vi "DEV test VIs wrapped.vi"() -> ()   [LabVIEW 2018, in "Image Management.lvlib"]
uses:
  Image Management.lvlib
  receipt parsing/Receipt Parsing.lvlib
  database/Items--cluster.ctl
  database/Database.lvlib
  database/Purchased_Items--cluster.ctl
  database/Visits--cluster.ctl
panel:
  out "TotalPrice":dbl
  out "Unit":string[](array[string])
  out "NumberOfUnits":dbl[](array[numeric])
  out "TaxStatus":string[](array[string])
  out "PrintedNames":string[](array[string])
  out "Prices":string[](array[string])
  out "Items":string[](array[string])
  out "Footer":string[](array[string])
  out "Header":string[](array[string])
  out "Main Body":string[](array[string])
  out "Image 2":T1(plugin-control)
  out "Array":string[](array[string])
  out "Columns (Pixels)":i32
  out "Rows (Pixels)":i32
  out "Image":T1(plugin-control)
  out "Rows Where Whitespace Starts":i32[](array[numeric])
  out "Image Pixels (I16)":i16[][](array[numeric])
  out "Error Out":errorcluster
  in  "Error In":errorcluster
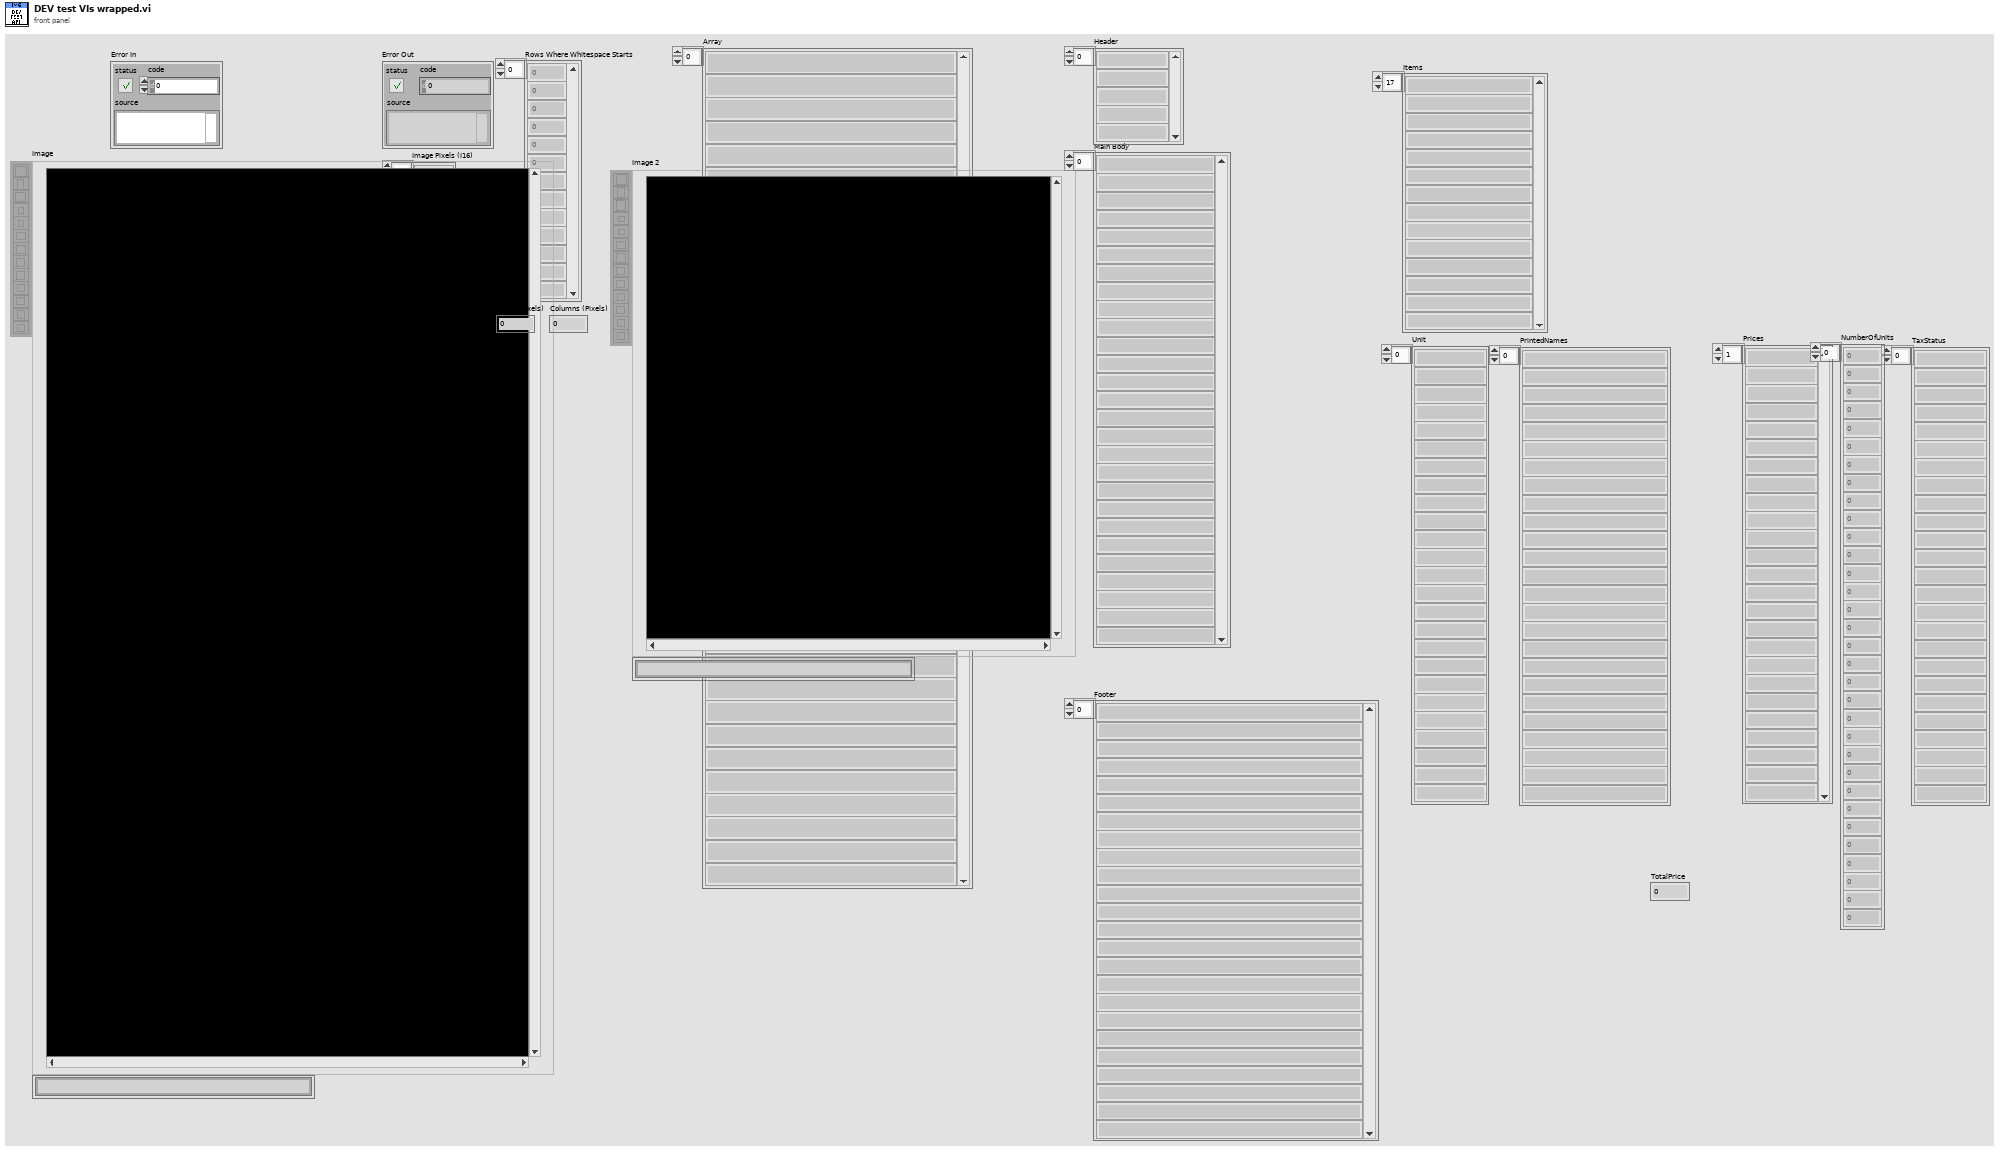
[diagram p1: front panel]
types:
  T1 = typedef "IMAQ Image.ctl" = refnum<image>
  T2 = typedef "Database.lvlib/Visits--cluster.ctl" = cluster{"Timestamp":timestamp, "TotalSpend":dbl, "SpendTaxedA":dbl, "SpendTaxedB":dbl, "Location":string, "NumberOfItems":i32, "NumberOfUniqueItems":i32, "TotalDiscount":dbl, "ReceiptImagePath":string}
  T3 = typedef "Database.lvlib/Purchased_Items--cluster.ctl" = cluster{"ItemName":string, "TotalPriceIncludingDiscount":dbl, "NumberOfUnits":i32, "VisitID":i32, "TotalDiscount":dbl}
  T4 = typedef "Database.lvlib/Items--cluster.ctl" = cluster{"ItemName":string, "PrintedNames":string, "TaxStatus":string, "Unit":string, "IsFood":bool, "IsVeg":bool, "IsFavourite":bool}
  T5 = typedef "ROI Descriptor" = cluster{"Global Rectangle":i32[], "Contours":cluster{"ID":enum32{"External", "Internal"}, "Type":u32, "Coordinates":i32[]}[]}
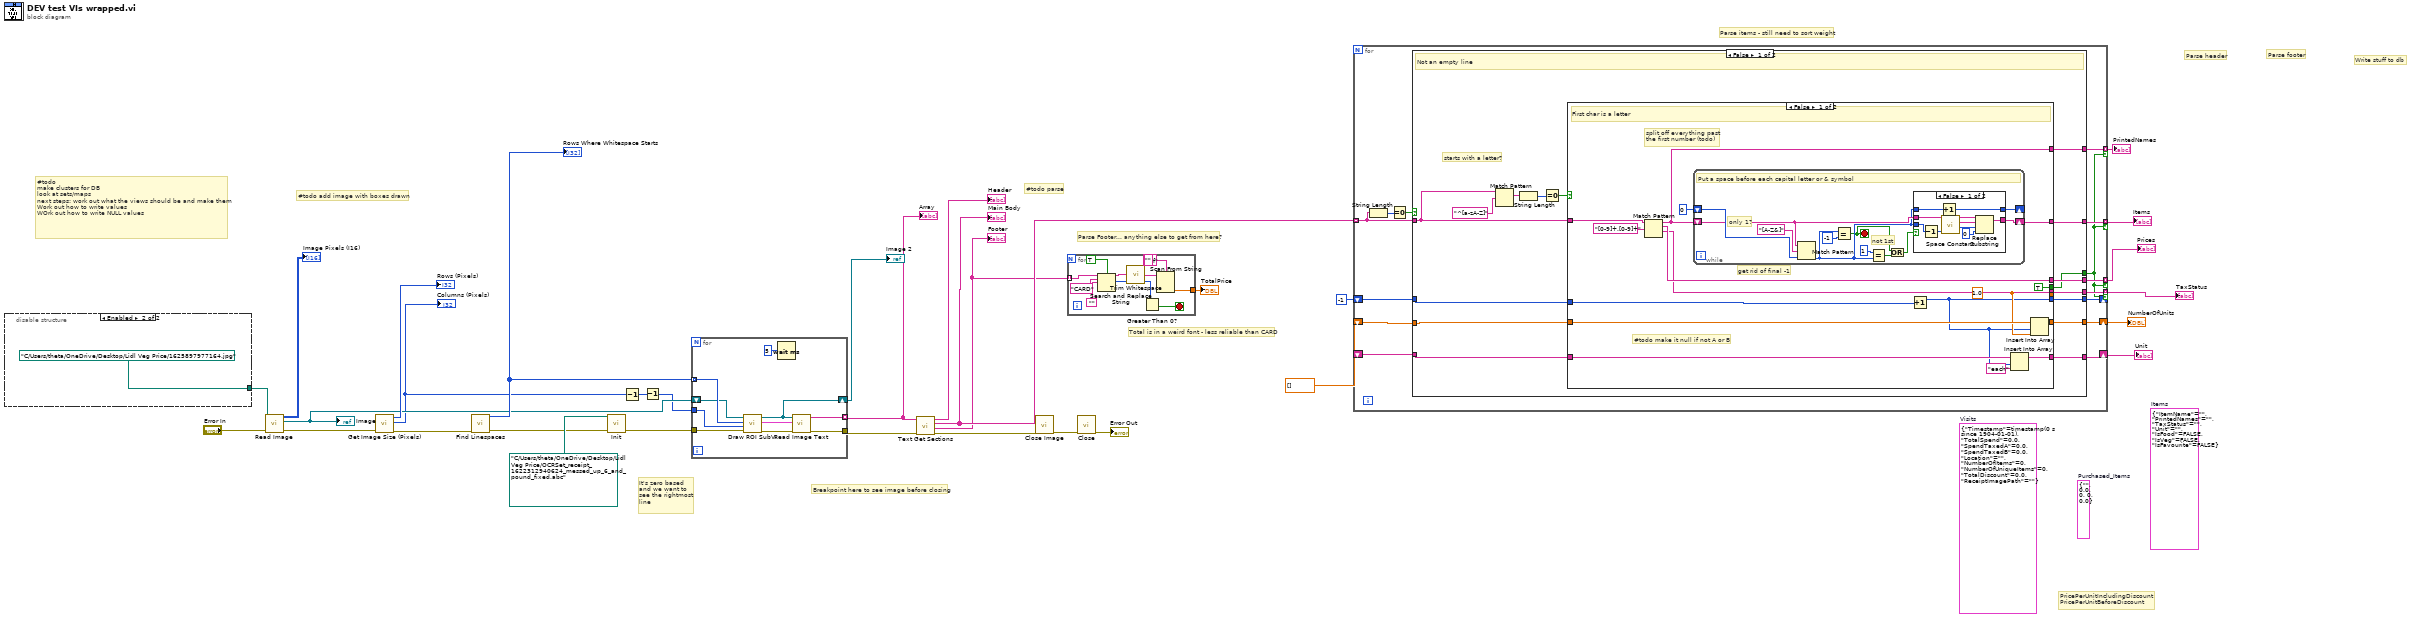
[diagram p0: block diagram]
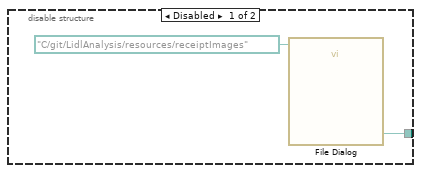
[diagram p2: hidden frame]
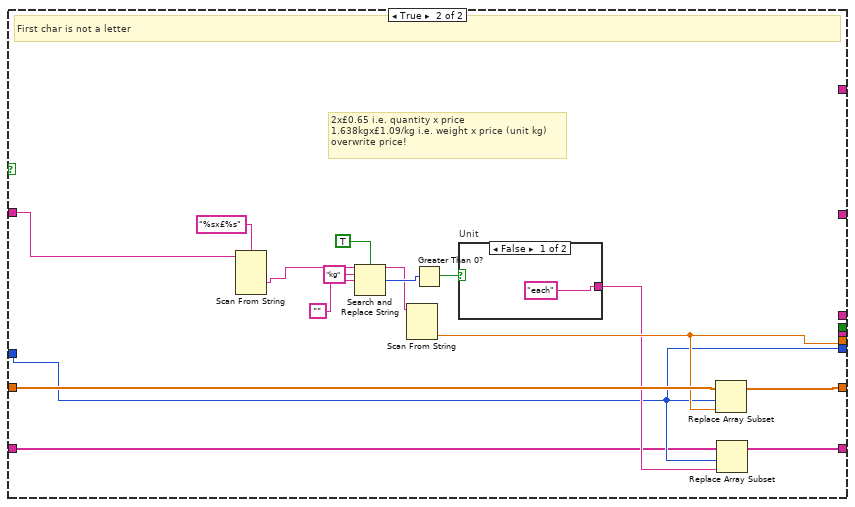
[diagram p4: hidden frame]
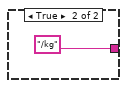
[diagram p5: hidden frame]
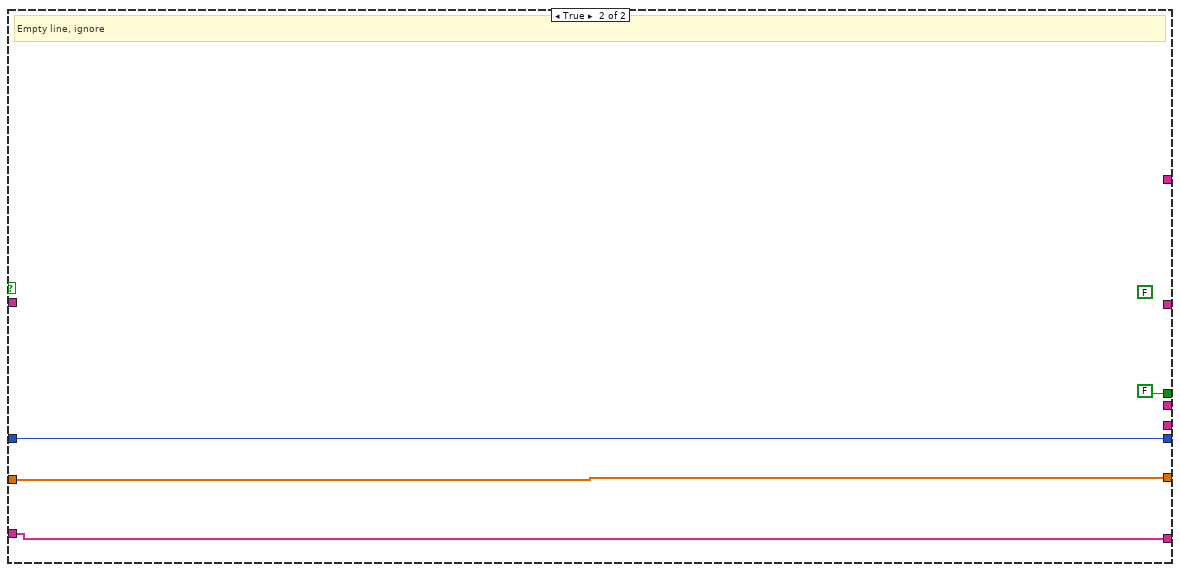
[diagram p6: hidden frame]
diagram:
  (unwired) T2 {"Timestamp"=timestamp(0 s since 1904-01-01), "TotalSpend"=0.0, "SpendTaxedA"=0.0, "SpendTaxedB"=0.0, "Location"="", "NumberOfItems"=0, "NumberOfUniqueItems"=0, "TotalDiscount"=0.0, "ReceiptImagePath"=""}  # Visits
  (unwired) T3 {"ItemName"="", "TotalPriceIncludingDiscount"=0.0, "NumberOfUnits"=0, "VisitID"=0, "TotalDiscount"=0.0}  # Purchased_Items
  (unwired) T4 {"ItemName"="", "PrintedNames"="", "TaxStatus"="", "Unit"="", "IsFood"=FALSE, "IsVeg"=FALSE, "IsFavourite"=FALSE}  # Items
  # "#todo\nmake clusters for DB\nlook at sets/maps\nnext steps: work out what the views should be and make them\nWork out how to write values\nWOrk out how to write NULL values"
  # "#todo parse"
  # "Parse Footer... anything else to get from here?"
  # "Total is in a weird font - less reliable than CARD"
  # "PricePerUnitIncludingDiscount\nPricePerUnitBeforeDiscount"
  # "Write stuff to db"
  # "Parse footer"
  # "Parse header"
  # "Parse items - still need to sort weight"
  # "Breakpoint here to see image before closing"
  # "It's zero based\nand we want to\nsee the rightmost\nline"
  # "#todo add image with boxes drawn"
  n1 = disable-structure shown="Enabled" {
    disable-tunnel: [w34 path "C:/Users/theta/OneDrive/Desktop/Lidl Veg Price/1625897977164.jpg" ("File Path")] -> w1
    frame Disabled {
      n2 = call "File Dialog"("start path"=path "C:/git/LidlAnalysis/resources/receiptImages") -> ("selected path"=w34:path)  [unwired: 11 in, 3 out]
    }
    frame Enabled {
    }
  }
  n3 = call "Read Image.vi"("Error In"="Error In", "File Path"=w1) -> ("Error Out"=w29:errorcluster, "Image"=w26:T1, "Image Pixels (I16)"=→"Image Pixels (I16)":u8[][])  [unwired: 7 in]
  "Image" <- w26
  n4 = call "Get Image Size (Pixels).vi"("Error In"=w29) -> ("Error Out"=w30:errorcluster, "Columns (Pixels)"=w25:i32, "Rows (Pixels)"=→"Rows (Pixels)":i32)  [unwired: 8 in]
  "Columns (Pixels)" <- w25
  n5 = call "Find Linespaces.vi"("error in (no error)"=w30) -> ("error out"=w17:errorcluster, "Rows where whitespace starts"=w27:i32[])  [unwired: 9 in]
  "Rows Where Whitespace Starts" <- w27
  n6 = call "Init.vi"("error in (no error)"=w17, "File Path"=path "C:/Users/theta/OneDrive/Desktop/Lidl Veg Price/OCRSet_receipt_1622312940624_messed_up_6_and_pound_fixed.abc") -> ("error out"=w18:errorcluster)  [unwired: 9 in]
  n7 = Decrement(x=w25) -> (x-1=w24:i32)
  n8 = Decrement(x=w24) -> (x-1=w23:i32)
  n9 = for {
    tunnel: w27 -> [w44] mode=indexing
    tunnel: w23 -> [w45]
    shift-right: [w37] -> w19
    shift-left: w26 -> [w43]
    tunnel: [w41] -> w13
    tunnel: [w40] -> w16 mode=indexing
    tunnel: w18 -> [w39]
    n10 = call "Draw ROI SubVI.vi"("error in (no error)"=w39, "Right Border location (pix)"=w45, "Horizontal Line location (pix)"=w44, "Refnum in"=w43) -> ("error out"=w38:errorcluster, "ROI Descriptor"=w36:T5, "Refnum out"=w37:T1)  [unwired: 5 in]
    n11 = Wait (ms)(milliseconds to wait=u32 5) -> ()  [unwired: 1 out]
    n12 = call "Read Image Text.vi"("Error In"=w38, "ROI Descriptor"=w36, "Image Ref"=w37) -> ("Error Out"=w41:errorcluster, "Line of Text"=w40:string)  [unwired: 7 in]
  }
  "Array" <- w16
  "Image 2" <- w19
  n13 = call "Text Get Sections.vi"("Error In"=w13, "Receipt Lines"=w16) -> ("Error Out"=w14:errorcluster, "Footer"=w3:string[], "Main Body"=w10:string[], "End of Header"=→"Header":string[])  [unwired: 5 in, 1 out]
  "Main Body" <- w10
  "Footer" <- w3
  n14 = call "Close Image.vi"("error in (no error)"=w14) -> ("error out"=w20:errorcluster)  [unwired: 10 in]
  n15 = for {
    tunnel: w3 -> [w55] mode=indexing
    tunnel: [w48] -> w2
    stop <- w47 stop-if-true
    (unwired) "%f" ("format string")
    n16 = Search and Replace String(case sensitive?=TRUE ("ignore case? (F)"), input string=w55, search string="CARD", replace string="") -> (result string=w51:string, number of replacements=w46:i32)  [unwired: 4 in, 2 out]
    n17 = call <vilib>:"Trim Whitespace.vi"("string"=w51) -> ("trimmed string"=w50:string)  [unwired: 1 in]
    n18 = Greater Than 0?(x=w46) -> (x > 0?=w47:bool)
    n19 = Scan From String(format string="", input string=w50) -> (output 1=w48:dbl)  [unwired: 3 in, 3 out]
  }
  "TotalPrice" <- w2
  n20 = call "Close.vi"("error in (no error)"=w20) -> ("error out"=→"Error Out":errorcluster)  [unwired: 10 in]
  n21 = for {
    tunnel: w10 -> [w67] mode=indexing
    tunnel: [w69] -> w12 mode=indexing if=w62
    tunnel: [w68] -> w11 mode=indexing if=w62
    tunnel: [w64] -> w9 mode=indexing if=w62
    tunnel: [w63] -> w8 mode=indexing if=w62
    shift-right: [w61] -> w7
    shift-left: dbl[] [] -> [w60]
    shift-right: [w58] -> _
    shift-left: -1 -> [w59]
    shift-right: [w57] -> w4
    shift-left: _ -> [w56]
    n22 = String Length(string=w67) -> (length=w66:i32)
    n23 = Equal To 0?(x=w66) -> (x = 0?=w65:bool)
    n24 = case shown="False" w65 {
      tunnel: [w85 _] -> w69
      tunnel: [w84 _] -> w68
      tunnel: w67 -> [w79 _]
      tunnel: [w78 FALSE] -> w62
      tunnel: [w77 _] -> w64
      tunnel: [w76 _] -> w63
      tunnel: [w73 w143] -> w61
      tunnel: w60 -> [w72 w143]
      tunnel: w59 -> [w74 w142]
      tunnel: [w75 w142] -> w58
      tunnel: [w71 w141] -> w57
      tunnel: w56 -> [w70 w141]
      frame False {
        # "starts with a letter?"
        # "Not an empty line"
        n25 = Match Pattern(string=w79, regular expression="^[a-zA-Z]") -> (match substring=w80:string)  [unwired: 1 in, 3 out]
        n26 = String Length(string=w80) -> (length=w83:i32)
        n27 = Equal To 0?(x=w83) -> (x = 0?=w82:bool)
        n28 = case shown="False" w82 {
          tunnel: w79 -> [w99 w138]
          tunnel: [w100 _] -> w85
          tunnel: [w97 _] -> w84
          tunnel: [TRUE _] -> w78
          tunnel: [w95 _] -> w77
          tunnel: [w94 _] -> w76
          tunnel: [w90 w127] -> _
          tunnel: [w87 w125] -> w75
          tunnel: w74 -> [w93 w125]
          tunnel: [w92 w128] -> w73
          tunnel: w72 -> [w91 w129]
          tunnel: [w89 w124] -> w71
          tunnel: w70 -> [w88 w123]
          frame False {
            w90 = 1.0
            # "#todo make it null if not A or B"
            # "split off everything past\nthe first number (todo)"
            # "get rid of final -1"
            # "First char is a letter"
            n29 = Match Pattern(string=w99, regular expression="[0-9]+.[0-9]+") -> (before substring=w95:string, match substring=w97:string, after substring=w94:string)  [unwired: 1 in, 1 out]
            n30 = while {
              shift-right: [w107] -> _
              shift-left: 0 ("offset past match") -> [w110]
              shift-right: [w109] -> w100
              shift-left: w95 -> [w108]
              stop <- w103 stop-if-true
              # "not 1st"
              # "only 1?"
              # "Put a space before each capital letter or & symbol"
              n31 = Match Pattern(string=w108, regular expression="[A-Z&]", offset (0)=w110) -> (offset past match=w105:i32)  [unwired: 3 out]
              n32 = Equal?(x=w105, y=-1) -> (x = y?=w103:bool)
              n33 = Equal?(x=1, y=w105) -> (x = y?=w106:bool)
              n34 = Or(x=w103, y=w106) -> (x .or. y?=w104:bool)
              n35 = case shown="False" w104 {
                tunnel: w105 -> [w117 _]
                tunnel: [w119 w122] -> w109
                tunnel: w108 -> [w118 w122]
                tunnel: w105 -> [w114 w121]
                tunnel: [w113 w121] -> w107
                frame False {
                  n36 = Decrement(x=w117) -> (x-1=w116:i32)
                  n37 = Increment(x=w114) -> (x+1=w113:i32)
                  n38 = call <vilib>:"Space Constant.vi"() -> ("String"=w120:string)
                  n39 = Replace Substring(2:0 ("length (len. of substring)"), 3:w116, 4:w120, 5:w118) -> (1:w119:string)  [unwired: 1 out]
                }
                frame True {
                }
              }
            }
            n40 = Increment(x=w93) -> (x+1=w87:i32)
            n41 = Insert Into Array(array=w88, index=w87, new element="each" ("new element/subarray")) -> (w89:string[])
            n42 = Insert Into Array(array=w91, index=w87, new element=w90) -> (w92:dbl[])
          }
          frame True {
            # "2x£0.65 i.e. quantity x price\n1.638kgx£1.09/kg i.e. weight x price (unit kg)\noverwrite price!"
            # "First char is not a letter"
            n43 = Scan From String(format string="%sx£%s", input string=w138) -> (output 1=w135:string)  [unwired: 5 in, 3 out]
            n44 = Search and Replace String(case sensitive?=TRUE ("ignore case? (F)"), input string=w135, search string="kg", replace string="") -> (result string=w130:string, number of replacements=w132:i32)  [unwired: 4 in, 2 out]
            n45 = Scan From String(input string=w130) -> (output 1=w127:dbl)  [unwired: 4 in, 3 out]
            n46 = Greater Than 0?(x=w132) -> (x > 0?=w133:bool)
            n47 = case "Unit" shown="False" w133 {
              tunnel: ["each" ("search string") "/kg" ("search string")] -> w126
              frame False {
              }
              frame True {
              }
            }
            n48 = Replace Array Subset(array=w129, new element=w127, index=w125) -> (w128:dbl[])
            n49 = Replace Array Subset(array=w123, new element=w126, index=w125) -> (w124:string[])
          }
        }
      }
      frame True {
        (unwired) FALSE
        # "Empty line, ignore"
      }
    }
  }
  "Items" <- w12
  "Prices" <- w11
  "PrintedNames" <- w9
  "TaxStatus" <- w8
  "NumberOfUnits" <- w7
  "Unit" <- w4
